vi "MemTest.vi"() -> ()   [LabVIEW 2012]
panel:
  in  "Data In":bool
  out "Data Out":bool
  out "F1":bool
  out "F2":bool
  out "CP":bool
  out "CT":bool
  in  "Slices":u32=2
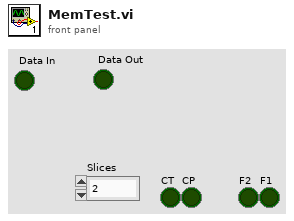
[diagram p1: front panel]
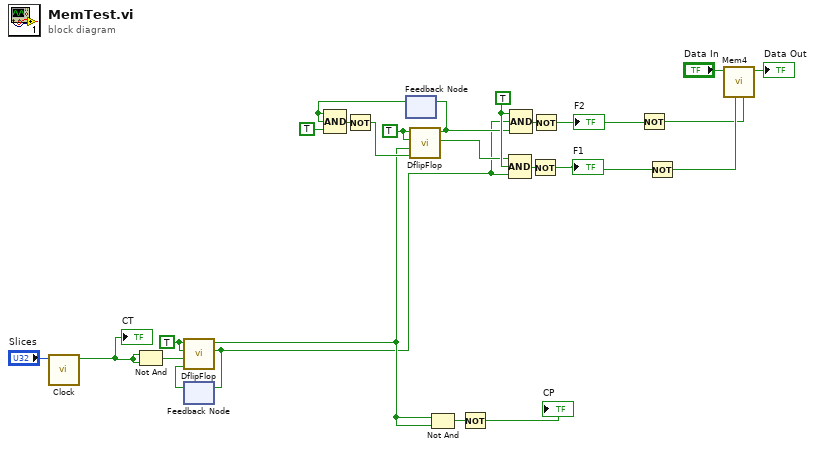
[diagram p0: block diagram]
diagram:
  w15 = TRUE
  w21 = TRUE ("Set")
  w23 = TRUE ("Set")
  n1 = call "Clock.vi"("Slices"="Slices") -> ("Clk"=w25:bool)  [unwired: 10 in]
  "CT" <- w25
  n2 = Not And(1:w25, 2:w25) -> (0:w24:bool)
  n3 = feedback #1() -> (w22:bool)  [unwired: 1 in]
  n4 = call "DflipFlop.vi"("D"=w22, "Clock"=w24, "Reset"=w23, "Set"=w23) -> ("/Q\\"=w8:bool, "Q"=w11:bool)  [unwired: 6 in]
  n5 = feedback-in #1(w8) -> ()
  n6 = feedback #2() -> (w18:bool)  [unwired: 1 in]
  n7 = Compound Arithmetic op=AND(w18, w18, TRUE ("value")) -> (w20:bool)
  n8 = Not(x=w20) -> (.not. x?=w19:bool)
  n9 = call "DflipFlop.vi"("D"=w19, "Clock"=w11, "Reset"=w21, "Set"=w21) -> ("/Q\\"=w14:bool, "Q"=w13:bool)  [unwired: 6 in]
  n10 = feedback-in #2(w13) -> ()
  n11 = Not And(1:w11, 2:w11) -> (0:w12:bool)
  n12 = Not(x=w12) -> (.not. x?=→"CP":bool)
  n13 = Compound Arithmetic op=AND(w14, w15, w8) -> (w16:bool)
  n14 = Compound Arithmetic op=AND(w15, w8, w13) -> (w17:bool)
  n15 = Not(x=w16) -> (.not. x?=w6:bool)
  "F1" <- w6
  n16 = Not(x=w17) -> (.not. x?=w4:bool)
  "F2" <- w4
  n17 = Not(x=w4) -> (.not. x?=w3:bool)
  n18 = Not(x=w6) -> (.not. x?=w5:bool)
  n19 = call "Mem4.vi"("Phi1"=w3, "Phi0"=w5, "Data In"="Data In") -> ("Data Out"=→"Data Out":bool)  [unwired: 8 in]
